vi "Normalize Phi.vi"(11 "phi":dbl) -> (3 "Phi":dbl)   [LabVIEW 2018]
panel:
  out "Target_Phi_end":dbl
  out "Target_Phi_1":dbl
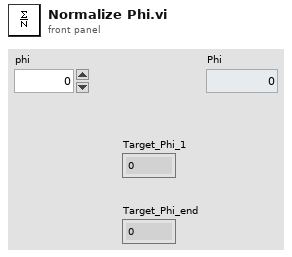
[diagram p1: front panel]
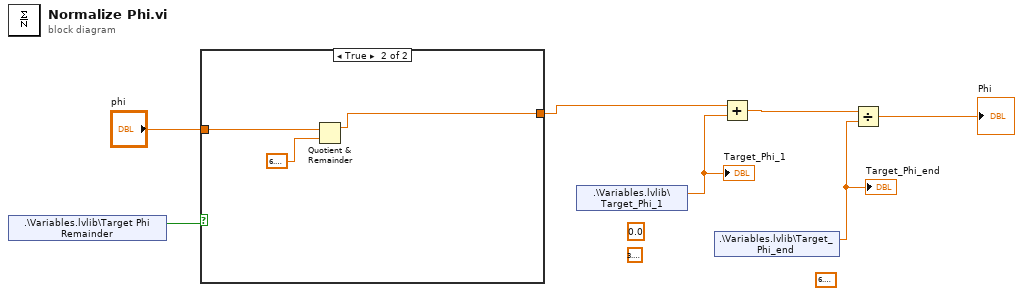
[diagram p0: block diagram]
diagram:
  (unwired) 0.0
  (unwired) 6.283185307179586
  (unwired) 3.141592653589793
  n1 = shared-variable ".\\Variables.lvlib\\Target Phi Remainder"() -> (w1:bool)  [unwired: 1 in, 1 out]
  n2 = case shown="True" w1 {
    tunnel: "phi" -> [w8 w11]
    tunnel: [w8 w10] -> w2
    frame False {
    }
    frame True {
      n3 = Quotient & Remainder(x=w11, y=6.283185307179586) -> (x-y*floor(x/y)=w10:dbl)  [unwired: 1 out]
    }
  }
  n4 = shared-variable ".\\Variables.lvlib\\Target_Phi_1"() -> (w5:dbl)  [unwired: 1 in, 1 out]
  "Target_Phi_1" <- w5
  n5 = shared-variable ".\\Variables.lvlib\\Target_Phi_end"() -> (w6:dbl)  [unwired: 1 in, 1 out]
  "Target_Phi_end" <- w6
  n6 = Add(x=w2, y=w5) -> (x+y=w7:dbl)
  n7 = Divide(x=w7, y=w6) -> (x/y=→"Phi":dbl)
